vi "Make single scan multivariable array file.vi"(10 "P(x)":dbl[][](array[numeric])=[[-1.74, 0.00227273], [1.07, -0.00113636]] caption="P(x) ascending order of power." min=0.0 max=127.0 format="%#.6f", 11 "Cluster":T2={"Scan parameters"={"Scan Start"=0.0, "Scan End"=22.0, "Scan Step Size"=4.0, "# Shots Each Step"=5, "single direction?"=TRUE}, "device and variable preamble"="Device = \"PL1-Hexapod,PL1-Hexapod,PL1-Hexapod\"\nVariable = \"xpos,ypos,zpos\""} {"Scan parameters"."Scan Start" format="%#.9p"; "Scan parameters"."Scan End" format="%#.9p"; "Scan parameters"."Scan Step Size" format="%#.9p"}) -> ()   [LabVIEW 2013]
uses:
  scan parameters.ctl
panel:
  in  "SaveConfig":bool
  in  "ReadConfig":bool
  in  "makescanstring":bool
  in  "OK":bool
  in  "precision primary":i16=2
  in  "precision other (12)":i16=4
  out "spreadsheet string":string="[Scan1]\r\nDevice = \"PL1-Hexapod,PL1-Hexapod,PL1-Hexapod\"\nVariable = \"xpos,ypos,zpos\"\r\nValues:#shots = \"(0.00,-1.7400,1.0700):5|(4.00,-1.7309,1.0655):5|(8.00,-1.7218,1.0609):5|(12.00,-1.7127,1.0564):5|(16.00,-1.7036,1.0518):5|(20.00,-1.6945,1.0473):5\""
  # "Instructions:\neg set device and variable preamble are... Device = \"PL1-PresCtrl-Low1,PlasmaLensLowPressureControl\"\nVariable = \"P. Control Up (Torr),pressure\""
  # "each row a set of polynomials\nshould match device and variable preampe"
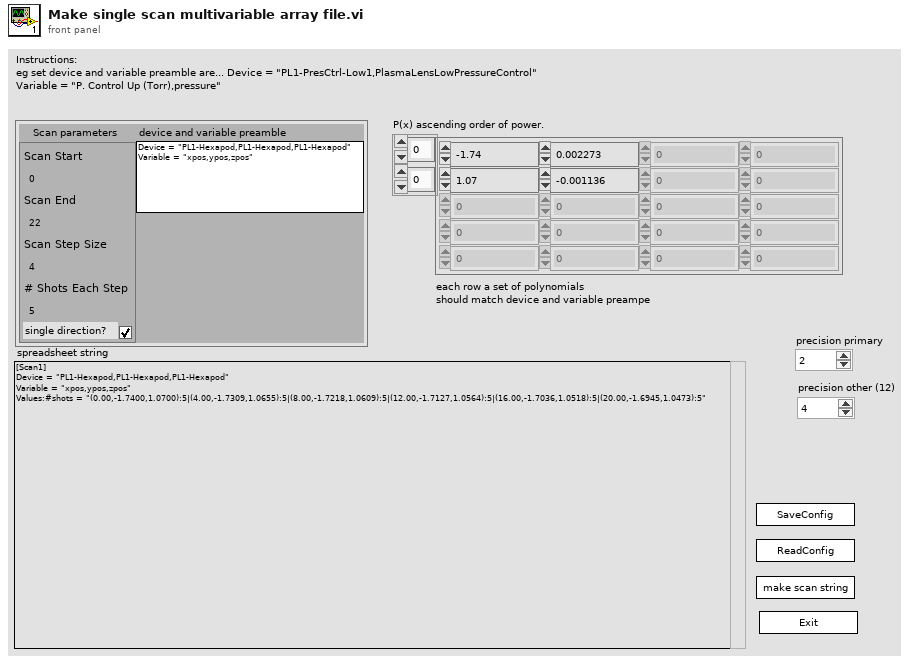
[diagram p1: front panel]
types:
  T1 = typedef "scan parameters.ctl" = cluster{"Scan Start":dbl, "Scan End":dbl, "Scan Step Size":dbl, "# Shots Each Step":u32, "single direction?":bool}
  T2 = cluster{"Scan parameters":T1, "device and variable preamble":string}
  T3 = enum32{"Invalid", "Standard", "Closed", "Hidden", "Minimized", "Maximized"}
  T4 = enum32{"invalid app kind", "Development System", "Run Time System", "Student Edition", "Embedded LabVIEW", "Evaluation", "Custom"}
  T5 = cluster{"Core":cluster{"Current VI Reference":refnum<vi>, "Close Panel on Exit?":bool}, "inputs":cluster{"precision primary 2":i16, "Cluster 2":cluster{"Scan parameters":T1, "device and variable preamble":string}, "P(x) 2":dbl[][], "precision other (12) 2":i16}, "Your string data":string}
  T6 = cluster{"precision primary 2":i16, "Cluster 2":cluster{"Scan parameters":T1, "device and variable preamble":string}, "P(x) 2":dbl[][], "precision other (12) 2":i16}
  T7 = cluster{"Current VI Reference":refnum<vi>, "Close Panel on Exit?":bool}
  T8 = cluster{"precision primary":i16, "Cluster":cluster{"Scan parameters":T1, "device and variable preamble":string}, "P(x)":dbl[][], "precision other (12)":i16}
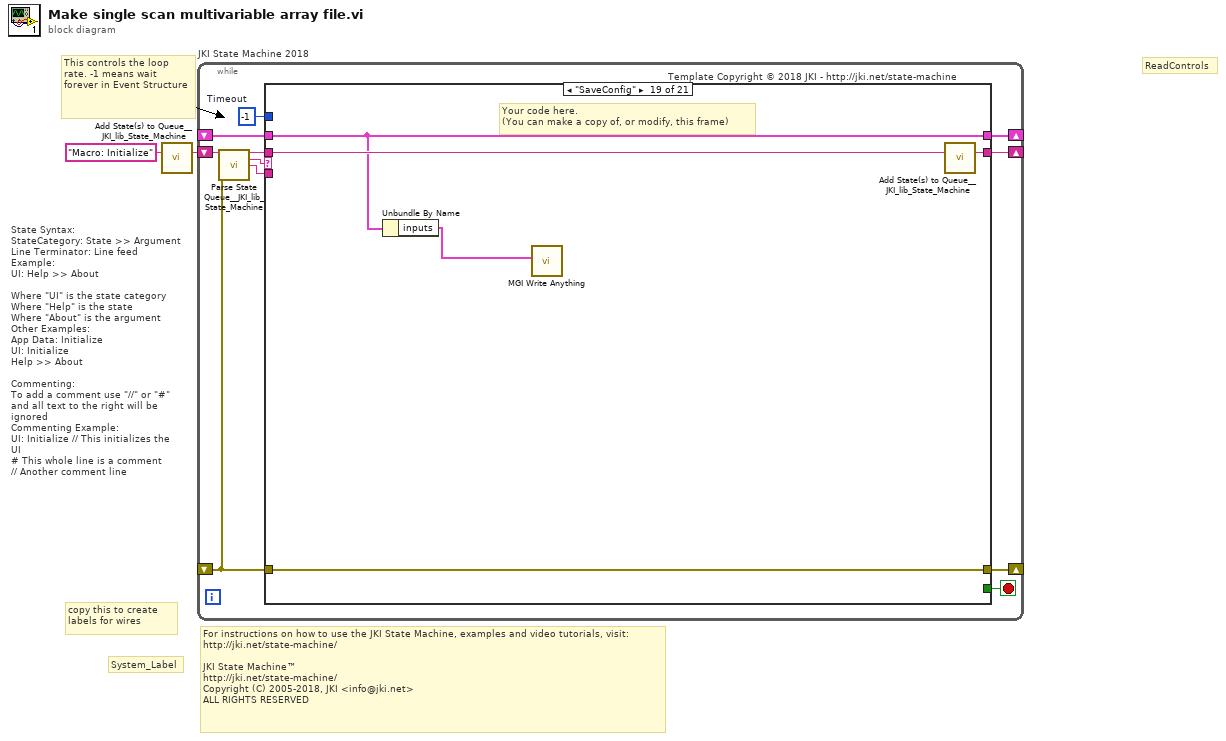
[diagram p0: block diagram]
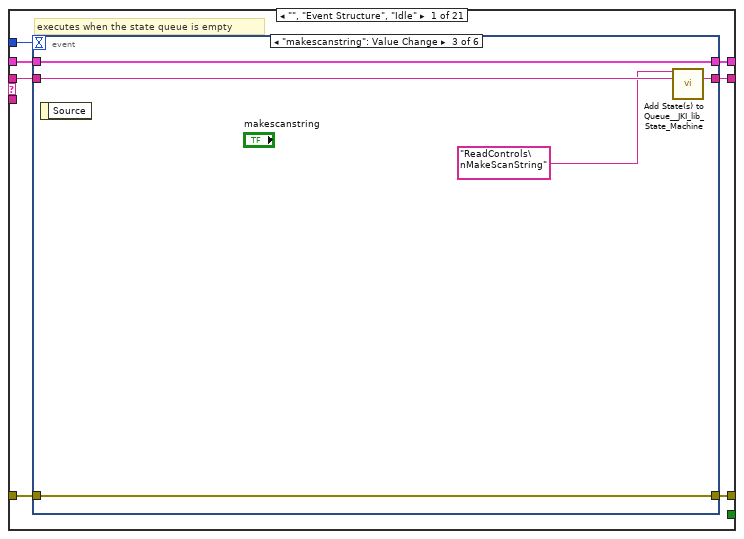
[diagram p2: hidden frame]
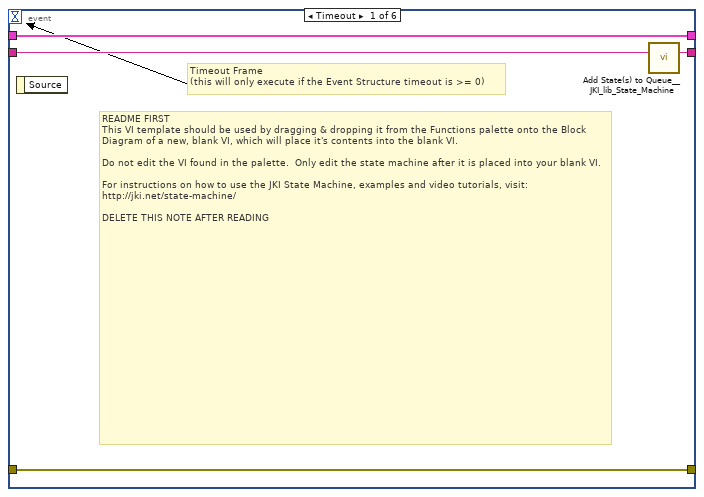
[diagram p3: hidden frame]
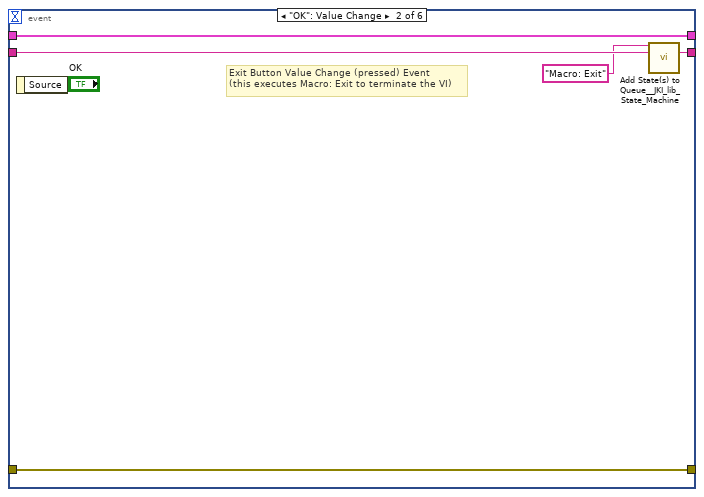
[diagram p4: hidden frame]
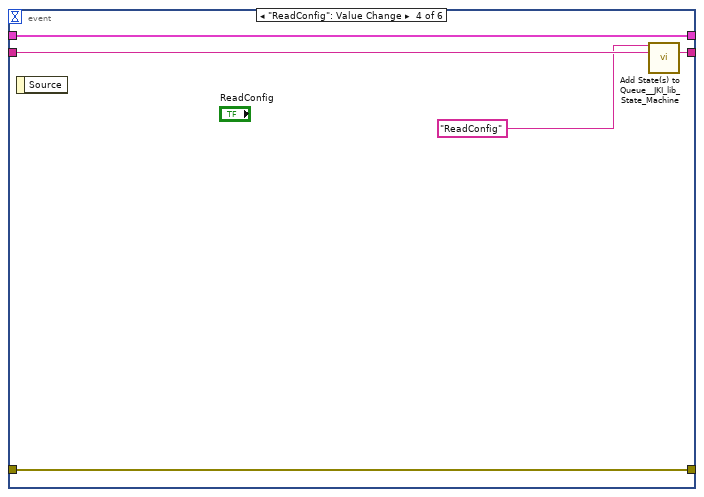
[diagram p5: hidden frame]
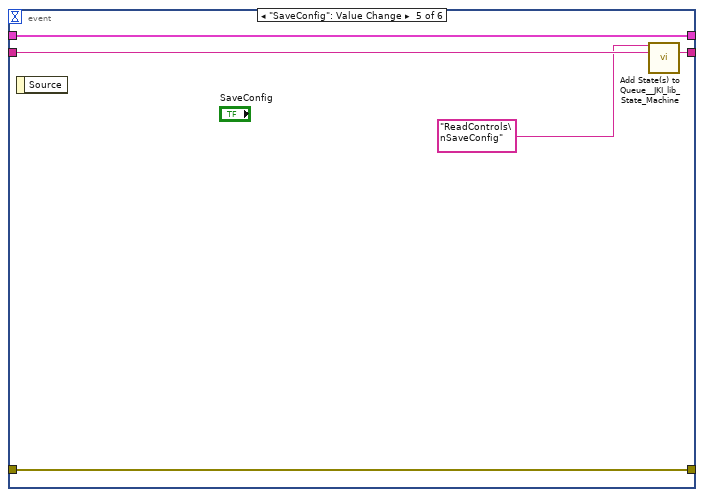
[diagram p6: hidden frame]
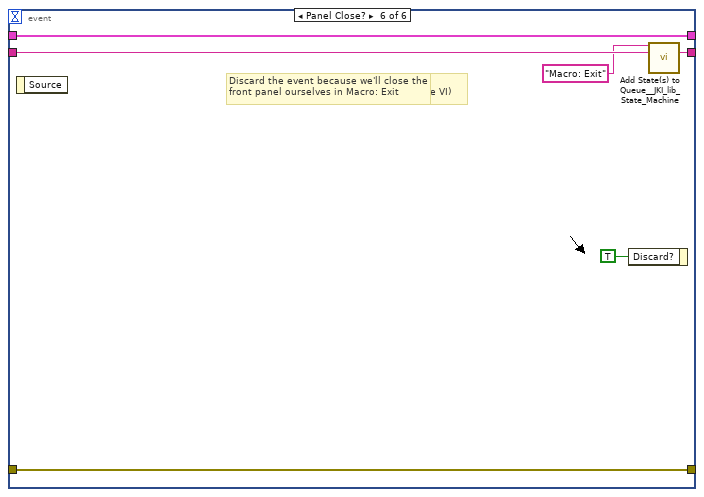
[diagram p7: hidden frame]
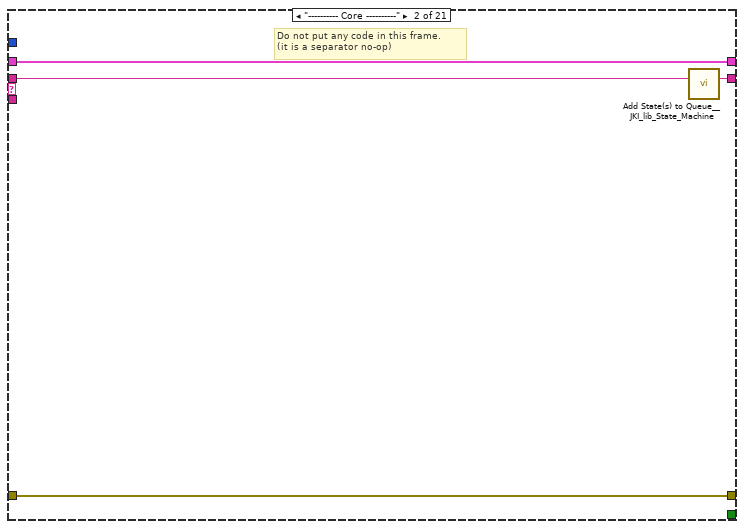
[diagram p8: hidden frame]
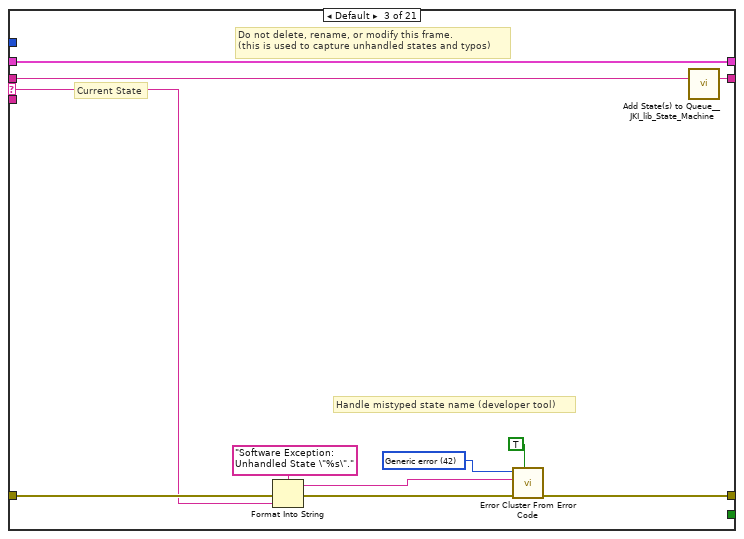
[diagram p9: hidden frame]
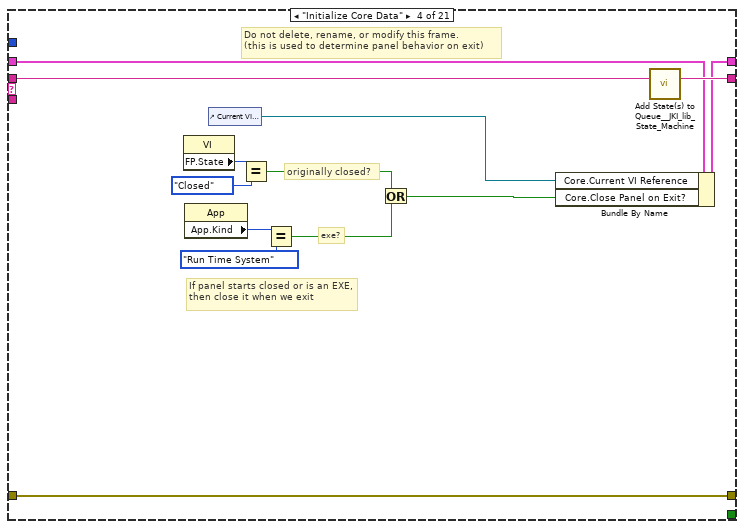
[diagram p10: hidden frame]
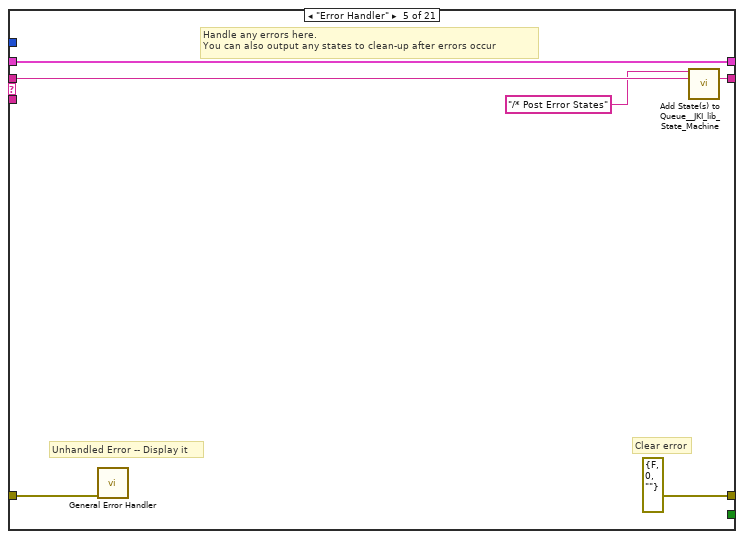
[diagram p11: hidden frame]
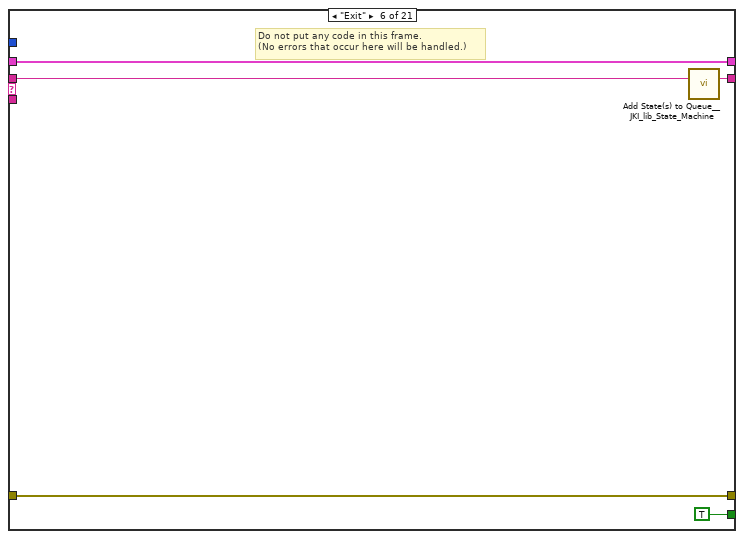
[diagram p12: hidden frame]
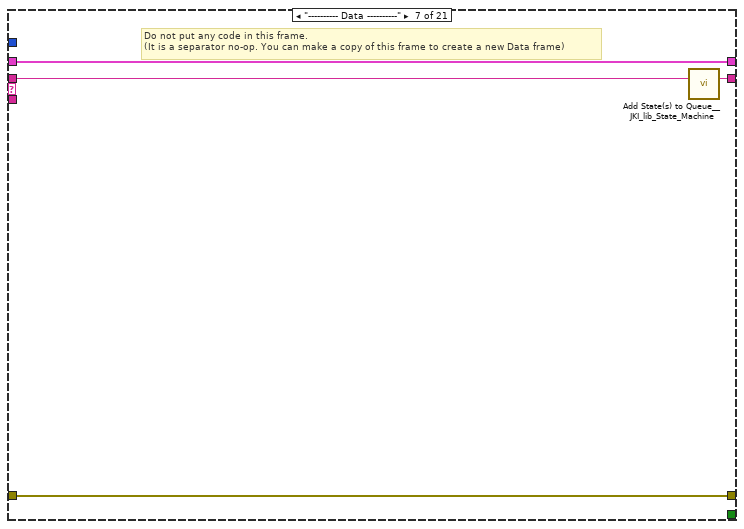
[diagram p13: hidden frame]
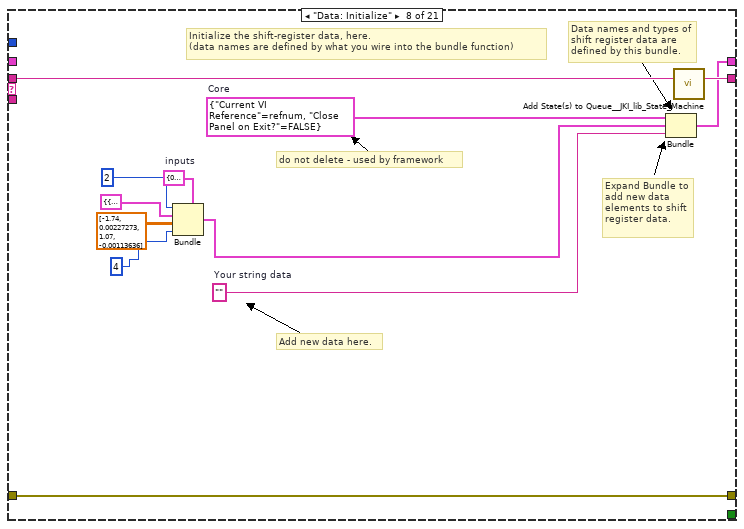
[diagram p14: hidden frame]
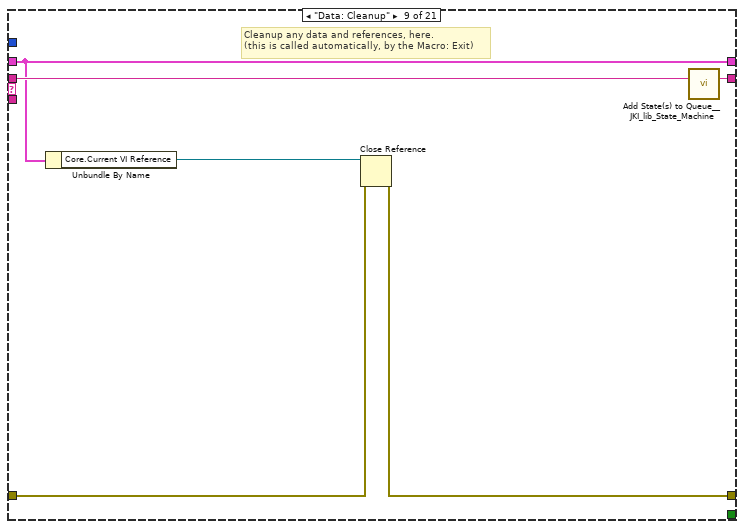
[diagram p15: hidden frame]
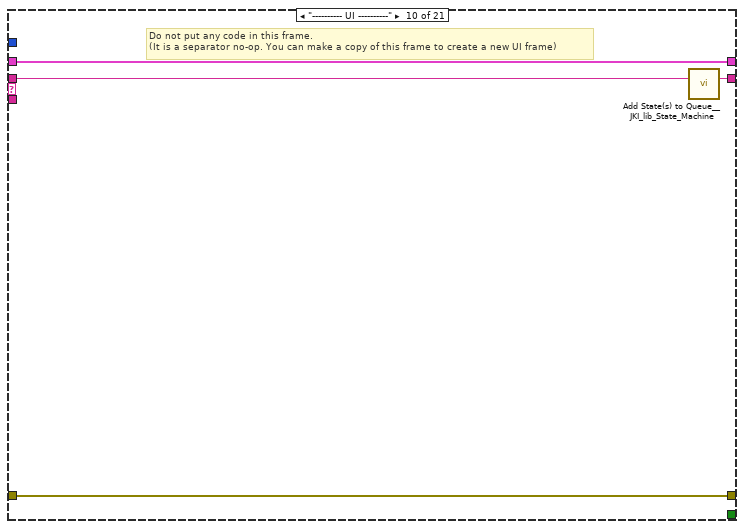
[diagram p16: hidden frame]
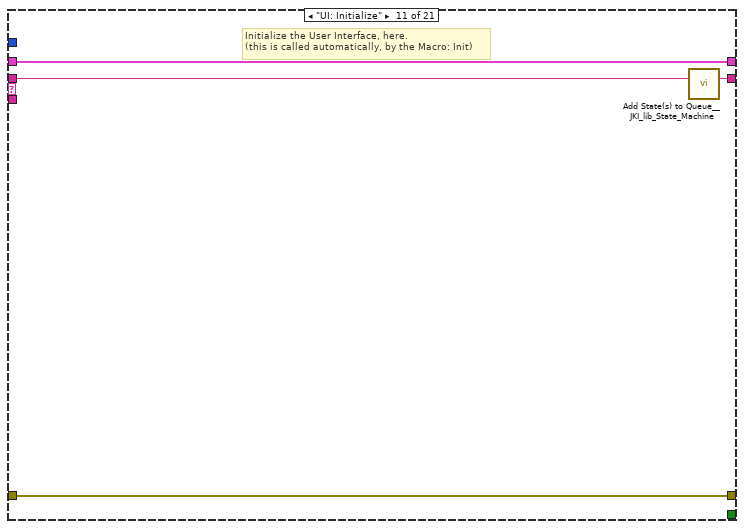
[diagram p17: hidden frame]
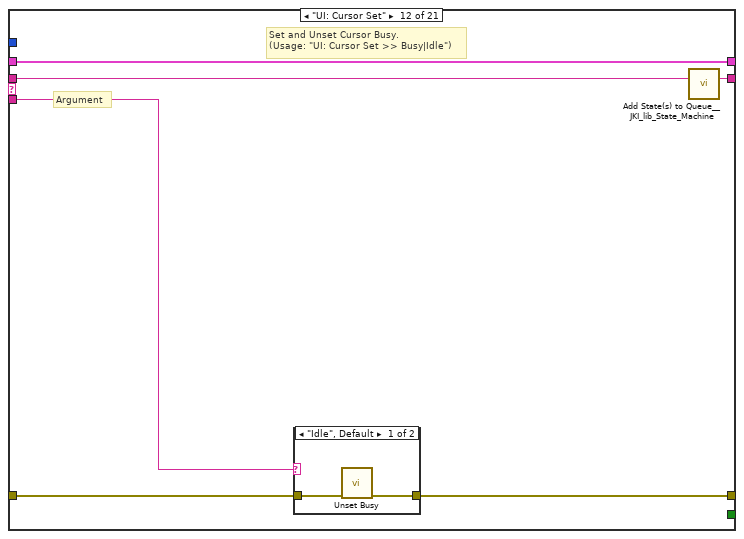
[diagram p18: hidden frame]
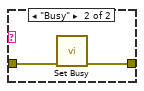
[diagram p19: hidden frame]
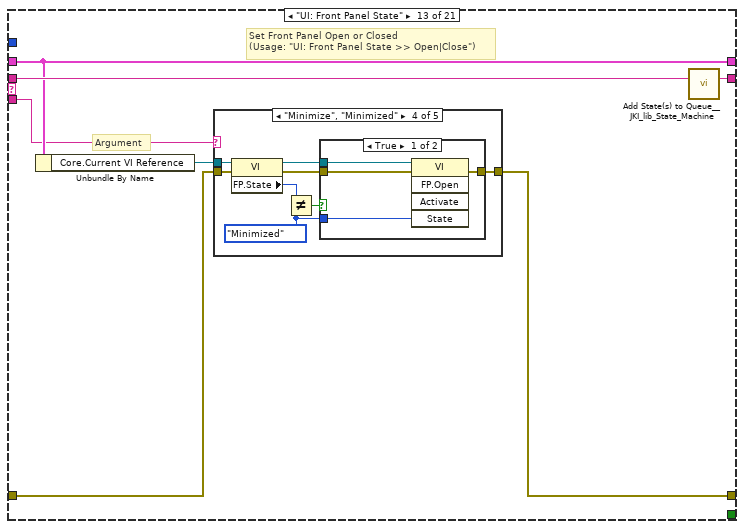
[diagram p20: hidden frame]
diagram:
  # "ReadControls"
  # "For instructions on how to use the JKI State Machine, examples and video tutorials, visit:\nhttp://jki.net/state-machine/\n\nJKI State Machine™\nhttp://jki.net/state-machine/\nCopyright (C) 2005-2018, JKI <info@jki.net>\nALL RIGHTS RESERVED"
  # "State Syntax:\nStateCategory: State >> Argument\nLine Terminator: Line feed\nExample:\nUI: Help >> About\n\nWhere \"UI\" is the state category\nWhere \"Help\" is the state\nWhere \"About\" is the argument\nOther Examples:\nApp Data: Initialize\nUI: Initialize\nHelp >> About\n\nCommenting:\nTo add a comment use \"//\" or \"#\" and all text to the right will be ignored\nCommenting Example:\nUI: Initialize // This initializes the UI\n# This whole line is a comment\n// Another comment line"
  # "copy this to create labels for wires"
  # "This controls the loop rate. -1 means wait forever in Event Structure"
  # "System_Label"
  n1 = call <vilib>:"Add State(s) to Queue__JKI_lib_State_Machine.vi"("State(s) in (\"\")"="Macro: Initialize") -> ("States Out"=w2:string)  [unwired: 14 in]
  n2 = while "JKI State Machine 2018" {
    shift-right: [w6] -> _
    shift-left: _ -> [w5]
    shift-right: [w9] -> _
    shift-left: _ -> [w3]
    shift-right: [w8] -> _
    shift-left: w2 -> [w10]
    stop <- w7 stop-if-true
    w4 = -1  # Timeout
    # "Template Copyright © 2018 JKI - http://jki.net/state-machine"
    n3 = call <vilib>:"Parse State Queue__JKI_lib_State_Machine.vi"("State Queue"=w10, "Error In (no error)"=w3) -> ("Remaining States"=w12:string, "Current State"=w13:string, "Arguments"=w11:string)  [unwired: 11 in]
    n4 = case shown="\"SaveConfig\"" w13 {
      selector: w13 -> [_ _ w55 _ _ _ _ _ _ _ _ _ _ _ _ _ _ _ _ _ _]
      tunnel: w12 -> [w20 w54 w59 w78 w84 w89 w93 w105 w111 w115 w119 w125 w136 w205 w210 w220 w224 w234 w239 w253 w262]
      tunnel: w11 -> [_ _ _ _ _ _ _ _ _ _ _ w120 w130 _ _ _ _ _ _ _ _]
      tunnel: w5 -> [w18 w51 w57 w71 w81 w87 w90 _ w106 w112 w117 w123 w132 w202 w207 w217 w221 w227 w236 w248 w258]
      tunnel: [w17 w52 w61 w75 errorcluster {"status"=FALSE, "code"=0, "source"=""} ("error out") w86 w91 w102 w107 w113 w116 w121 w133 w203 w208 w218 w222 w232 w237 w245 w260] -> w9
      tunnel: w3 -> [w16 w52 w60 w75 w80 w86 w91 w102 w108 w113 w116 w122 w134 w203 w208 w218 w222 w232 w237 w246 w260]
      tunnel: [w19 w53 w58 w77 w83 w88 w92 w104 w110 w114 w118 w124 w135 w204 w209 w219 w223 w233 w238 w252 w261] -> w8
      tunnel: [_ _ _ _ _ TRUE _ _ _ _ _ _ _ _ _ _ _ _ _ _ _] -> w7
      tunnel: [w15 w51 w57 w76 w81 w87 w90 w103 w106 w112 w117 w123 w132 w202 w207 w217 w221 w226 w236 w247 w258] -> w6
      tunnel: w4 -> [w14 _ _ _ _ _ _ _ _ _ _ _ _ _ _ _ _ _ _ _ _]
      frame "", "Event Structure", "Idle" {
        # "executes when the state queue is empty"
        n5 = event shown="[2] \"makescanstring\": Value Change" {
          selector: _ -> [_ _ _ _ _ _]
          dyn-events: _ -> [_ _ _ _ _ _]
          timeout: w14 -> [_ _ _ _ _ _]
          tunnel: w20 -> [w24 w29 w34 w39 w44 w50]
          tunnel: [w23 w28 w33 w38 w43 w49] -> w19
          tunnel: w18 -> [w21 w26 w31 w36 w41 w47]
          tunnel: [w22 w27 w32 w37 w42 w48] -> w17
          tunnel: w16 -> [w22 w27 w32 w37 w42 w48]
          tunnel: [w21 w26 w31 w36 w41 w47] -> w15
          event Timeout {
            # "README FIRST\nThis VI template should be used by dragging & dropping it from the Functions palette onto the Block Diagram of a new, blank VI, which will place it's contents into the blank VI.\n\nDo not edit the VI found in the palette.  Only edit the state machine after it is placed into your blank VI.\n\nFor instructions on how to use the JKI State Machine, examples and video tutorials, visit:\nhttp://jki.net/state-machine/\n\nDELETE THIS NOTE AFTER READING"
            # "Timeout Frame\n(this will only execute if the Event Structure timeout is >= 0)"
            n6 = event-data() -> ()  [unwired: 1 in, 1 out]
            n7 = call <vilib>:"Add State(s) to Queue__JKI_lib_State_Machine.vi"("State(s) in (\"\")"=w24) -> ("States Out"=w23:string)  [unwired: 14 in]
          }
          event "OK": Value Change {
            # "Exit Button Value Change (pressed) Event\n(this executes Macro: Exit to terminate the VI)"
            n8 = event-data() -> ()  [unwired: 1 in, 1 out]
            n9 = call <vilib>:"Add State(s) to Queue__JKI_lib_State_Machine.vi"("State(s) in Front (\"\")"="Macro: Exit", "State(s) in (\"\")"=w29) -> ("States Out"=w28:string)  [unwired: 13 in]
          }
          event "makescanstring": Value Change {
            n10 = event-data() -> ()  [unwired: 1 in, 1 out]
            n11 = call <vilib>:"Add State(s) to Queue__JKI_lib_State_Machine.vi"("State(s) in Front (\"\")"="ReadControls\nMakeScanString", "State(s) in (\"\")"=w34) -> ("States Out"=w33:string)  [unwired: 13 in]
          }
          event "ReadConfig": Value Change {
            n12 = event-data() -> ()  [unwired: 1 in, 1 out]
            n13 = call <vilib>:"Add State(s) to Queue__JKI_lib_State_Machine.vi"("State(s) in Front (\"\")"="ReadConfig", "State(s) in (\"\")"=w39) -> ("States Out"=w38:string)  [unwired: 13 in]
          }
          event "SaveConfig": Value Change {
            n14 = event-data() -> ()  [unwired: 1 in, 1 out]
            n15 = call <vilib>:"Add State(s) to Queue__JKI_lib_State_Machine.vi"("State(s) in Front (\"\")"="ReadControls\nSaveConfig", "State(s) in (\"\")"=w44) -> ("States Out"=w43:string)  [unwired: 13 in]
          }
          event Panel Close? {
            # "Discard the event because we'll close the front panel ourselves in Macro: Exit"
            # "Close Panel button (pressed) Event\n(this executes Macro: Exit to terminate the VI)"
            n16 = event-data() -> ()  [unwired: 1 in, 1 out]
            n17 = event-data("Discard?"=TRUE) -> ()  [unwired: 1 in, 1 out]
            n18 = call <vilib>:"Add State(s) to Queue__JKI_lib_State_Machine.vi"("State(s) in Front (\"\")"="Macro: Exit", "State(s) in (\"\")"=w50) -> ("States Out"=w49:string)  [unwired: 13 in]
          }
        }
      }
      frame "---------- Core ----------" {
        # "Do not put any code in this frame.\n(it is a separator no-op)"
        n19 = call <vilib>:"Add State(s) to Queue__JKI_lib_State_Machine.vi"("State(s) in (\"\")"=w54) -> ("States Out"=w53:string)  [unwired: 14 in]
      }
      frame Default {
        w64 = 42 items=["No error", "Argument error", "Memory is full", "Out of zone", "End of file", "File already open", "Generic file I/O error", "File not found", "File permission error", "Disk is full", "Duplicate path", "Too many files open", "System feature not enabled", "Resource file not found", "Cannot add resource", "Resource not found", "Image not found", "Image memory error", "Pen does not exist", "Config type invalid", "Config token not found", "Config parse error", "Config memory error", "Bad external code format", "Bad external code offset", "External code not present", "Null window", "Destroy window error", "Null menu", "Print aborted", "Bad print record", "Print driver error", "Windows error during printing", "Memory error during printing", "Print dialog error", "Generic print error", "Invalid device refnum", "Device not found", "Device parameter error", "Device unit error", "Cannot open device", "Device call aborted", "Generic error", "Cancelled by user", "Object ID too low", "Object ID too high", "Object not in heap", "Unknown heap", "Unknown object (invalid DefProc)", "Unknown object (DefProc not in table)", "Message out of range", "Invalid (null) method", "Unknown message", "Manager call not supported", "Bad address", "Network operation in progress", "Network operation timed out", "Connection is busy", "Network attribute not supported", "Network error", "Address in use", "System out of memory", "Connection aborted", "Connection refused", "Not connected", "Already connected", "Connection closed", "Initialization error (interapplication manager)", "Bad occurrence", "Wait on unbound occurrence handler", "Occurrence queue overflow", "Datalog type conflict", "Unused", "Unrecognized type (interapplication manager)", "Memory corrupt", "Failed to make temporary DLL", "Old CIN version", "Drag socket not found", "Failed to load drop-object", "Failed to register OLE object", "Failed to release OLE object", "Format specifier type mismatch", "Unknown format specifier", "Too few format specifiers", "Too many format specifiers", "Scan failed", "Newer CIN version", "Error converting to variant", "Runtime menu error", "Password tampered", "Variant attribute not found", "Incompatible variant data type", "Event data is not available", "Event Store is not present", "Occurrence is not found", "Event Queue is not created", "Event info is not available", "Refnum passed is NULL", "Error retrieving Class GUID", "Error retrieving CoClass GUID", "Error retrieving TypeLib GUID.", "Bad built application magic bytes.", "Specific driver is different from the specific driver associated with the Logical Name.", "There is no session opened to the class driver.", "Max Error", "MAX - Error with config objects", "MAX - Error loading configuration", "MAX - Group not supported"]
        # "Current State"
        # "Do not delete, rename, or modify this frame.\n(this is used to capture unhandled states and typos)"
        # "Handle mistyped state name (developer tool)"
        n20 = Format Into String(format string="Software Exception: Unhandled State \"%s\"." ("message"), error in=w60, w55) -> (resulting string=w63:string, error out=w62:errorcluster)  [unwired: 1 in]
        n21 = call <vilib>:"Error Cluster From Error Code.vi"("show call chain? (False)"=TRUE, "error in (no error)"=w62, "error message (\"\")"=w63, "error code (0)"=w64) -> ("error out"=w61:errorcluster)  [unwired: 5 in]
        n22 = call <vilib>:"Add State(s) to Queue__JKI_lib_State_Machine.vi"("State(s) in (\"\")"=w59) -> ("States Out"=w58:string)  [unwired: 14 in]
      }
      frame "Initialize Core Data" {
        # "Do not delete, rename, or modify this frame.\n(this is used to determine panel behavior on exit)"
        # "originally closed?"
        # "exe?"
        # "If panel starts closed or is an EXE, then close it when we exit"
        n23 = property class="VI"() -> ("FP.State"=w68:T3)  [unwired: 2 in, 2 out]
        n24 = property class="App"() -> ("App.Kind"=w74:T4)  [unwired: 2 in, 2 out]
        n25 = control-ref of="Current VI Reference"() -> (w69:refnum<vi>)
        n26 = Equal?(x=w68, y=T3."Closed" ("Front Panel Window:State")) -> (x = y?=w66:bool)
        n27 = Equal?(x=w74, y=T4."Run Time System" ("Application:Kind")) -> (x = y?=w72:bool)
        n28 = Or(x=w66, y=w72) -> (x .or. y?=w70:bool)
        n29 = Bundle By Name(cluster=w71, "Core.Current VI Reference"=w69, "Core.Close Panel on Exit?"=w70) -> (w76:T5)
        n30 = call <vilib>:"Add State(s) to Queue__JKI_lib_State_Machine.vi"("State(s) in (\"\")"=w78) -> ("States Out"=w77:string)  [unwired: 14 in]
      }
      frame "Error Handler" {
        # "Unhandled Error -- Display it"
        # "Handle any errors here.\nYou can also output any states to clean-up after errors occur"
        # "Clear error"
        n31 = call <vilib>:"General Error Handler.vi"("error in (no error)"=w80) -> ()  [unwired: 10 in, 5 out]
        n32 = call <vilib>:"Add State(s) to Queue__JKI_lib_State_Machine.vi"("State(s) in Front (\"\")"="/* Post Error States", "State(s) in (\"\")"=w84) -> ("States Out"=w83:string)  [unwired: 13 in]
      }
      frame "Exit" {
        # "Do not put any code in this frame.\n(No errors that occur here will be handled.)"
        n33 = call <vilib>:"Add State(s) to Queue__JKI_lib_State_Machine.vi"("State(s) in (\"\")"=w89) -> ("States Out"=w88:string)  [unwired: 14 in]
      }
      frame "---------- Data ----------" {
        # "Do not put any code in this frame.\n(It is a separator no-op. You can make a copy of this frame to create a new Data frame)"
        n34 = call <vilib>:"Add State(s) to Queue__JKI_lib_State_Machine.vi"("State(s) in (\"\")"=w93) -> ("States Out"=w92:string)  [unwired: 14 in]
      }
      frame "Data: Initialize" {
        w94 = T6 {"precision primary 2"=0, "Cluster 2"={"Scan parameters"={"Scan Start"=0.0, "Scan End"=0.0, "Scan Step Size"=0.0, "# Shots Each Step"=0, "single direction?"=FALSE}, "device and variable preamble"=""}, "P(x) 2"=[], "precision other (12) 2"=0}  # inputs
        w100 = T7 {"Current VI Reference"=refnum, "Close Panel on Exit?"=FALSE}  # Core
        w101 = ""  # Your string data
        # "do not delete - used by framework"
        # "Expand Bundle to add new data elements to shift register data."
        # "Add new data here."
        # "Data names and types of shift register data are defined by this bundle."
        # "Initialize the shift-register data, here.\n(data names are defined by what you wire into the bundle function)"
        n35 = Bundle(cluster=w94, "precision primary 2"=i16 2, "Cluster 2"=T2 {"Scan parameters"={"Scan Start"=0.0, "Scan End"=22.0, "Scan Step Size"=4.0, "# Shots Each Step"=5, "single direction?"=TRUE}, "device and variable preamble"="Device = \"PL1-Hexapod,PL1-Hexapod,PL1-Hexapod\"\nVariable = \"xpos,ypos,zpos\""}, "P(x) 2"=dbl[][] [[-1.74, 0.00227273], [1.07, -0.00113636]], "precision other (12) 2"=i16 4) -> (w95:T6)
        n36 = Bundle("Core"=w100, "inputs"=w95, "Your string data"=w101) -> (w103:T5)  [unwired: 1 in]
        n37 = call <vilib>:"Add State(s) to Queue__JKI_lib_State_Machine.vi"("State(s) in (\"\")"=w105) -> ("States Out"=w104:string)  [unwired: 14 in]
      }
      frame "Data: Cleanup" {
        # "Cleanup any data and references, here.\n(this is called automatically, by the Macro: Exit)"
        n38 = Unbundle By Name(w106) -> ("Core.Current VI Reference"=w109:refnum<vi>)
        n39 = Close Reference(reference=w109, error in (no error)=w108) -> (error out=w107:errorcluster)
        n40 = call <vilib>:"Add State(s) to Queue__JKI_lib_State_Machine.vi"("State(s) in (\"\")"=w111) -> ("States Out"=w110:string)  [unwired: 14 in]
      }
      frame "---------- UI ----------" {
        # "Do not put any code in this frame.\n(It is a separator no-op. You can make a copy of this frame to create a new UI frame)"
        n41 = call <vilib>:"Add State(s) to Queue__JKI_lib_State_Machine.vi"("State(s) in (\"\")"=w115) -> ("States Out"=w114:string)  [unwired: 14 in]
      }
      frame "UI: Initialize" {
        # "Initialize the User Interface, here.\n(this is called automatically, by the Macro: Init)"
        n42 = call <vilib>:"Add State(s) to Queue__JKI_lib_State_Machine.vi"("State(s) in (\"\")"=w119) -> ("States Out"=w118:string)  [unwired: 14 in]
      }
      frame "UI: Cursor Set" {
        # "Argument"
        # "Set and Unset Cursor Busy.\n(Usage: \"UI: Cursor Set >> Busy|Idle\")"
        n43 = case shown="\"Idle\", Default" w120 {
          tunnel: w122 -> [w127 w129]
          tunnel: [w126 w128] -> w121
          frame "Idle", Default {
            n44 = call <vilib>:"Unset Busy.vi"("error in (no error)"=w127) -> ("error out"=w126:errorcluster)  [unwired: 10 in]
          }
          frame "Busy" {
            n45 = call <vilib>:"Set Busy.vi"("error in (no error)"=w129) -> ("error out"=w128:errorcluster)  [unwired: 9 in, 1 out]
          }
        }
        n46 = call <vilib>:"Add State(s) to Queue__JKI_lib_State_Machine.vi"("State(s) in (\"\")"=w125) -> ("States Out"=w124:string)  [unwired: 14 in]
      }
      frame "UI: Front Panel State" {
        # "Argument"
        # "Set Front Panel Open or Closed\n(Usage: \"UI: Front Panel State >> Open|Close\")"
        n47 = Unbundle By Name(w132) -> ("Core.Current VI Reference"=w131:refnum<vi>)
        n48 = case shown="\"Minimize\", \"Minimized\"" w130 {
          tunnel: w134 -> [w142 w157 w168 w181 w194]
          tunnel: [w144 w158 w170 w183 w196] -> w133
          tunnel: w131 -> [w143 w155 w169 w182 w195]
          frame "Open", "Standard", Default {
            w137 = T3."Standard" ("State")
            n49 = property class="VI"(reference=w143, error in=w142) -> (reference out=w140:refnum<vi>, error out=w141:errorcluster, "FP.State"=w139:T3)
            n50 = Not Equal?(x=w139, y=w137) -> (x != y?=w138:bool)
            n51 = case shown="True" w138 {
              tunnel: [w148 w150] -> w144
              tunnel: w141 -> [w147 w150]
              tunnel: w140 -> [w146 _]
              tunnel: w137 -> [w145 _]
              frame True {
                n52 = invoke class="VI" method="FP.Open"(reference=w146, error in=w147, "Activate"=TRUE, "State"=w145) -> (error out=w148:errorcluster)  [unwired: 1 in, 4 out]
              }
              frame False {
              }
            }
          }
          frame "Close", "Closed" {
            n53 = property class="VI"(reference=w155, error in=w157) -> (reference out=w154:refnum<vi>, error out=w156:errorcluster, "FP.State"=w152:T3)
            n54 = Not Equal?(x=w152, y=T3."Closed" ("Front Panel Window:State")) -> (x != y?=w151:bool)
            n55 = case shown="True" w151 {
              tunnel: [w159 w162] -> w158
              tunnel: w156 -> [w159 w161]
              tunnel: w154 -> [_ w160]
              frame False {
              }
              frame True {
                n56 = invoke class="VI" method="FP.Close"(reference=w160, error in=w161) -> (error out=w162:errorcluster)  [unwired: 1 in, 2 out]
              }
            }
          }
          frame "Hidden", "Hide" {
            w163 = T3."Hidden" ("State")
            n57 = property class="VI"(reference=w169, error in=w168) -> (reference out=w166:refnum<vi>, error out=w167:errorcluster, "FP.State"=w165:T3)
            n58 = Not Equal?(x=w165, y=w163) -> (x != y?=w164:bool)
            n59 = case shown="True" w164 {
              tunnel: [w174 w175] -> w170
              tunnel: w167 -> [w173 w175]
              tunnel: w166 -> [w172 _]
              tunnel: w163 -> [w171 _]
              frame True {
                n60 = invoke class="VI" method="FP.Open"(reference=w172, error in=w173, "State"=w171) -> (error out=w174:errorcluster)  [unwired: 2 in, 4 out]
              }
              frame False {
              }
            }
          }
          frame "Minimize", "Minimized" {
            w176 = T3."Minimized" ("State")
            n61 = property class="VI"(reference=w182, error in=w181) -> (reference out=w179:refnum<vi>, error out=w180:errorcluster, "FP.State"=w178:T3)
            n62 = Not Equal?(x=w178, y=w176) -> (x != y?=w177:bool)
            n63 = case shown="True" w177 {
              tunnel: [w187 w188] -> w183
              tunnel: w180 -> [w186 w188]
              tunnel: w179 -> [w185 _]
              tunnel: w176 -> [w184 _]
              frame True {
                n64 = invoke class="VI" method="FP.Open"(reference=w185, error in=w186, "State"=w184) -> (error out=w187:errorcluster)  [unwired: 2 in, 4 out]
              }
              frame False {
              }
            }
          }
          frame "Maximize", "Maximized" {
            w189 = T3."Maximized" ("State")
            n65 = property class="VI"(reference=w195, error in=w194) -> (reference out=w192:refnum<vi>, error out=w193:errorcluster, "FP.State"=w191:T3)
            n66 = Not Equal?(x=w191, y=w189) -> (x != y?=w190:bool)
            n67 = case shown="True" w190 {
              tunnel: [w200 w201] -> w196
              tunnel: w193 -> [w199 w201]
              tunnel: w192 -> [w198 _]
              tunnel: w189 -> [w197 _]
              frame True {
                n68 = invoke class="VI" method="FP.Open"(reference=w198, error in=w199, "State"=w197) -> (error out=w200:errorcluster)  [unwired: 2 in, 4 out]
              }
              frame False {
              }
            }
          }
        }
        n69 = call <vilib>:"Add State(s) to Queue__JKI_lib_State_Machine.vi"("State(s) in (\"\")"=w136) -> ("States Out"=w135:string)  [unwired: 14 in]
      }
      frame "---------- Macro ----------" {
        # "Do not put any code in this frame.\n(It is a separator no-op. You can make a copy of this frame to create a new Macro frame)"
        n70 = call <vilib>:"Add State(s) to Queue__JKI_lib_State_Machine.vi"("State(s) in (\"\")"=w205) -> ("States Out"=w204:string)  [unwired: 14 in]
      }
      frame "Macro: Initialize" {
        w206 = "Data: Initialize\nInitialize Core Data\nUI: Initialize\nUI: Front Panel State >> Open"  # Data: Initialize Initialize Core Data UI: Initialize UI: Front Panel State >> Open
        # "Initialization Macro\n(This is called once, when the VI starts)"
        n71 = call <vilib>:"Add State(s) to Queue__JKI_lib_State_Machine.vi"("State(s) in Front (\"\")"=w206, "State(s) in (\"\")"=w210) -> ("States Out"=w209:string)  [unwired: 13 in]
      }
      frame "Macro: Exit" {
        # "Exit Macro\n(This is called once, when the VI exits)"
        n72 = Unbundle By Name(w217) -> ("Core.Close Panel on Exit?"=w216:bool)
        n73 = Select(t="UI: Front Panel State >> Close", s=w216, f="") -> (s? t:f=w213:string)
        n74 = call <vilib>:"Add State(s) to Queue__JKI_lib_State_Machine.vi"("State(s) in (\"\")"=w213, "State(s) at Back (\"\")"="Data: Cleanup\nExit") -> ("States Out"=w211:string)  [unwired: 13 in]
        n75 = call <vilib>:"Add State(s) to Queue__JKI_lib_State_Machine.vi"("State(s) in Front (\"\")"=w211, "State(s) in (\"\")"=w220) -> ("States Out"=w219:string)  [unwired: 13 in]
      }
      frame "---------- New Category ----------" {
        # "Template Separator\n(You can make a copy of, or modify, this frame)"
        n76 = call <vilib>:"Add State(s) to Queue__JKI_lib_State_Machine.vi"("State(s) in (\"\")"=w224) -> ("States Out"=w223:string)  [unwired: 14 in]
      }
      frame "ReadControls" {
        n77 = Bundle("precision primary"="precision primary", "Cluster"="Cluster", "P(x)"="P(x)", "precision other (12)"="precision other (12)") -> (w225:T8)  [unwired: 1 in]
        n78 = Bundle By Name(cluster=w227, "inputs"=w225) -> (w226:T5)
        n79 = call <vilib>:"Add State(s) to Queue__JKI_lib_State_Machine.vi"("State(s) in (\"\")"=w234) -> ("States Out"=w233:string)  [unwired: 14 in]
      }
      frame "SaveConfig" {
        # "Your code here.\n(You can make a copy of, or modify, this frame)"
        n80 = Unbundle By Name(w236) -> ("inputs"=w235:T6)
        n81 = call <userlib>:"MGI Write Anything.vi"("Anything"=w235) -> ()  [unwired: 8 in, 3 out]
        n82 = call <vilib>:"Add State(s) to Queue__JKI_lib_State_Machine.vi"("State(s) in (\"\")"=w239) -> ("States Out"=w238:string)  [unwired: 14 in]
      }
      frame "ReadConfig" {
        n83 = Unbundle By Name(w248) -> ("inputs"=w249:T6)
        n84 = call <userlib>:"MGI Read Anything.vi"("Type of Anything"=w249, "Error In"=w246) -> ("Error Out"=w250:errorcluster, "Anything"=w251:variant)  [unwired: 6 in, 2 out]
        n85 = Variant To Data(error in=w250, type=w249, Variant=w251) -> (data=w244:T6, error out=w245:errorcluster)
        n86 = Bundle By Name(cluster=w248, "inputs"=w244) -> (w247:T5)
        n87 = Unbundle(w244) -> ("precision primary 2"=w243:i16, "Cluster 2"=w242:T2, "P(x) 2"=w241:dbl[][], "precision other (12) 2"=w240:i16)
        n88 = local write "precision primary"(w243) -> ()
        n89 = local write "precision other (12)"(w240) -> ()
        n90 = local write "Cluster"(w242) -> ()
        n91 = local write "P(x)"(w241) -> ()
        n92 = call <vilib>:"Add State(s) to Queue__JKI_lib_State_Machine.vi"("State(s) in (\"\")"=w253) -> ("States Out"=w252:string)  [unwired: 14 in]
      }
      frame "MakeScanString" {
        n93 = Unbundle By Name(w258) -> ("inputs.precision primary 2"=w257:i16, "inputs.Cluster 2"=w256:T2, "inputs.P(x) 2"=w255:dbl[][], "inputs.precision other (12) 2"=w254:i16)
        n94 = call "make single scan multivariable array string.vi"("precision other (12)"=w254, "P(x)"=w255, "Cluster"=w256, "precision primary"=w257) -> ("String"=w259:string)  [unwired: 7 in]
        "spreadsheet string" <- w259
        n95 = disable-structure shown="Enabled" {
          disable-tunnel: w259 -> [w263 _]
          frame Enabled {
            n96 = call "File Dialog"() -> ("selected path"=w264:path, "error out"=w265:errorcluster)  [unwired: 12 in, 2 out]
            n97 = case shown="No Error" w265 {
              tunnel: w263 -> [w267 _]
              tunnel: w264 -> [w266 _]
              frame No Error {
                n98 = Write to Text File(file (use dialog)=w266, text=w267) -> ()  [unwired: 2 in, 3 out]
              }
              frame Error {
              }
            }
          }
          frame Disabled {
          }
        }
        n99 = call <vilib>:"Add State(s) to Queue__JKI_lib_State_Machine.vi"("State(s) in (\"\")"=w262) -> ("States Out"=w261:string)  [unwired: 14 in]
      }
    }
  }
